vi "STAGE+mono+counter_edit19.vi"() -> ()   [LabVIEW 2017]
panel:
  out "PROGRESS":u8(slide) max=10 step=10 scale=0.0..100.0
  in  "?":enum32{"Page 1", "Page 2"}(tab)
  out "XY Graph":cluster{dbl[], dbl[]}(graph)
  out "XY Graph 2":cluster{dbl[], dbl[]}[](graph)
  in  "Collect Data!":bool
  out "Timeout":bool
  in  "?":bool
  out "Timeout 2":bool
  out "Waveform Graph":waveform(dbl)[](graph)
  in  "?":enum32{"DELAY", "COUNTER", "MONO", "PLOT"}(tab)
  out "Final time [ps]":dbl
  out "Current time [ps]":dbl
  out "Initial time [ps]":dbl
  in  "Set this as t0":bool
  in  "Axis":i32=1
  in  "Motor ON":bool
  in  "Motor OFF":bool
  out "Current Position [mm]":dbl
  out "Final Position [mm]":dbl
  in  "Data Points":i32=100
  out "Current Point":i32
  in  "Step Size [um]":i32=10
  in  "Target [mm]":dbl format="%.3f"
  in  "Move":bool
  out "Initial position [mm]":dbl
  in  "GPIB address":string="23"
  in  "Count Mode":u16(ring) items=["A,B for Preset T", "A-B for Preset T", "A+B for Preset T", "A for Preset B"]
  in  "Trigger mode":u16(ring) items=["10 MHz"=0, "Input 2"=2, "Input T"=3]
  in  "Channel A Input":u16(ring)=1 items=["10 MHz", "Input 1"]
  in  "Channel B Input":u16(ring)=2 items=["Input 1"=1, "Input 2"=2]
  in  "Number of Measurements\n to take at one point/ Number of Periods":u16=1 min=1 max=2000 step=1
  in  "Time between measurements\n at one point (s)/Dwell Time":dbl=0.002 min=0.002 max=60.0 step=0.001
  in  "gate mode (CW:0)":i16(slide) scale=0.0..2.0 scale format="%.2f"
  out "Counts":i32
  in  "Integrating time \nin 10^-7 sec":dbl=10000000.0
  in  "Discriminator Level (mV)":dbl min=-300.0 max=300.0 step=0.2
  in  "Discriminator Slope":bool
  in  "Channel":i16 min=0 max=2 step=1
  out "Grating #":dbl
  out "Blaze angle":dbl
  out "Grooves/mm":dbl
  out "Mono port":T1(ring)
  out "Time delay":u32=450000 min=1
  in  "Step size":dbl=10.0 min=0.0
  in  "Scan to":i32=4000
  in  "Scan from":i32=2600
  out "Current wavelength":dbl
  in  "?":bool
  in  "Array":dbl[](array[numeric])
  out "Numeric":i32
  out "Numeric 2":i32
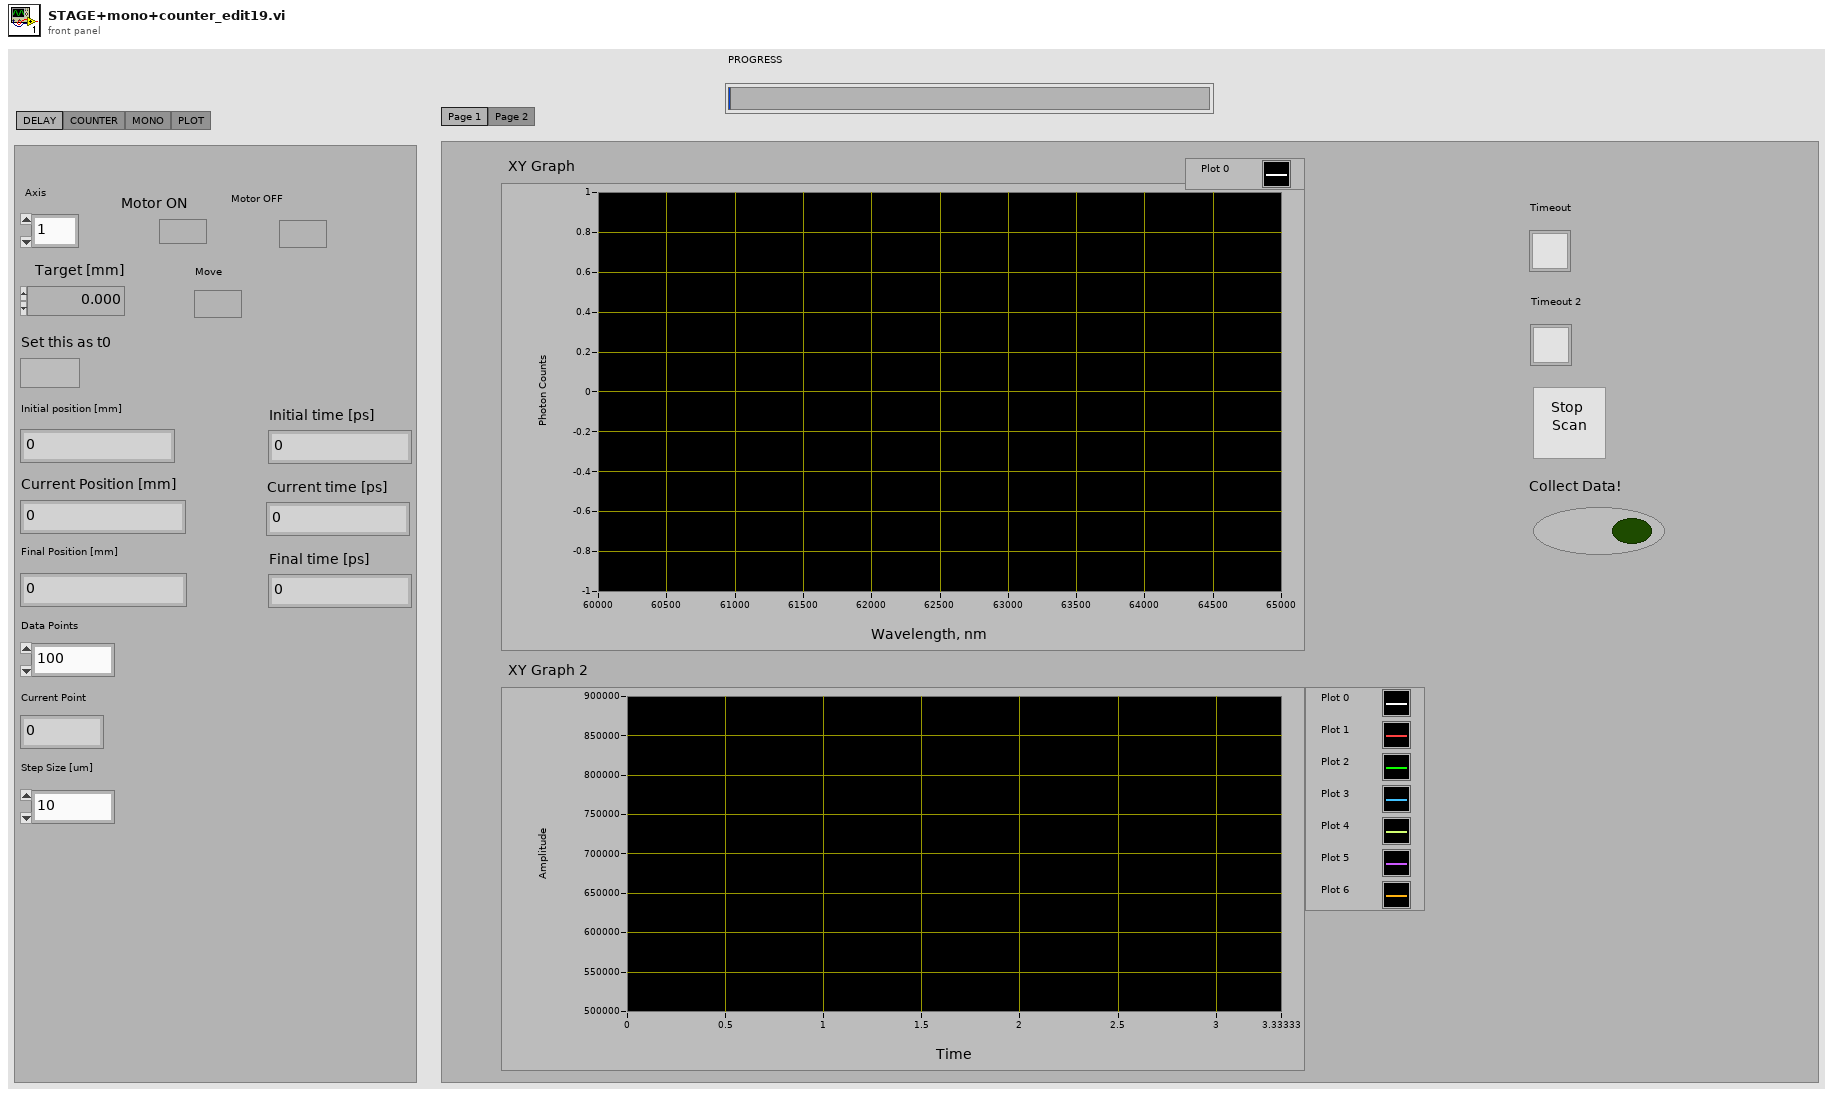
[diagram p1: front panel]
types:
  T1 = enum8{"COM 1", "COM 2", "COM 3", "COM 4", "COM 5", "COM 6", "COM 7", "COM 8", "COM 9"}
  T2 = cluster{"input XON/XOFF":bool, "input HW Handshake":bool, "input alt HW HShk":bool, "output XON/XOFF":bool, "output HW Handshake":bool, "output alt HW HShk":bool, "XOFF byte":u8, "XON byte":u8, "parity error byte":u16}
  T3 = enum16{"no parity", "odd parity", "even parity", "mark parity", "space parity"}
  T4 = typedef "NI_Matrix.lvlib/RealMatrix.ctl" = dbl[][]
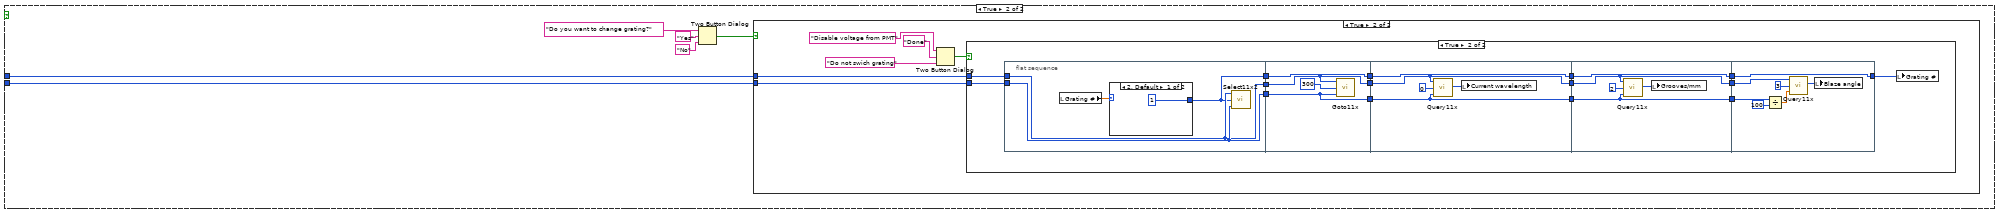
[diagram p2: hidden frame]
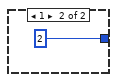
[diagram p5: hidden frame]
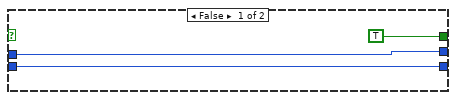
[diagram p6: hidden frame]
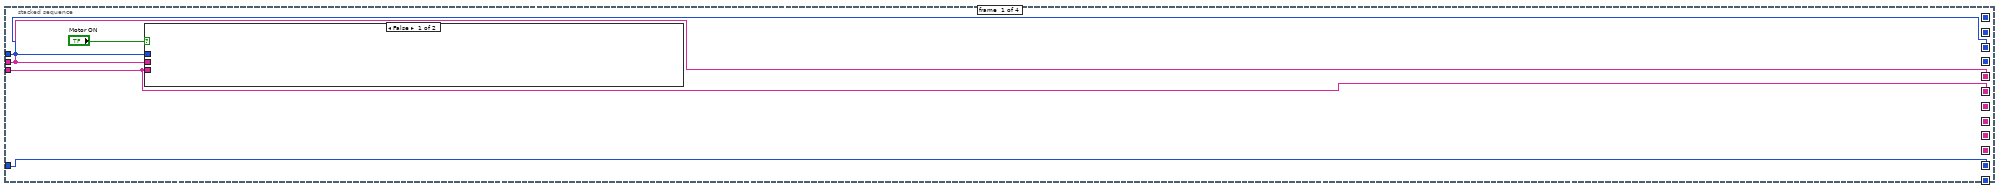
[diagram p7: hidden frame]
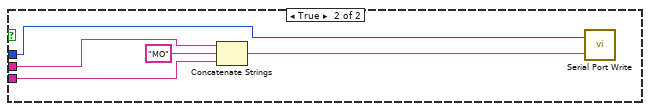
[diagram p8: hidden frame]
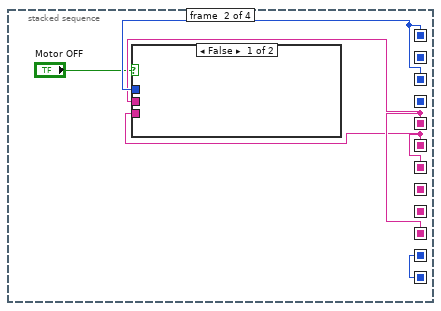
[diagram p9: hidden frame]
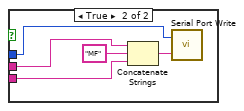
[diagram p10: hidden frame]
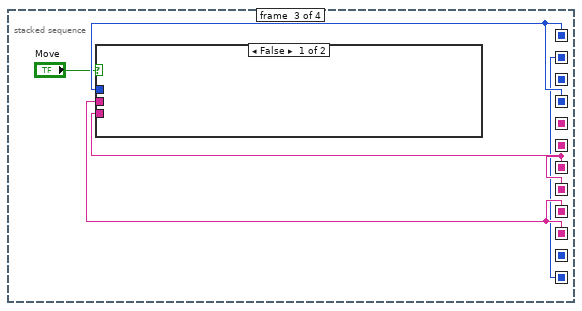
[diagram p11: hidden frame]
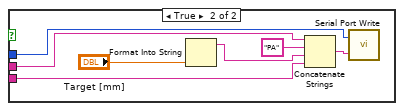
[diagram p12: hidden frame]
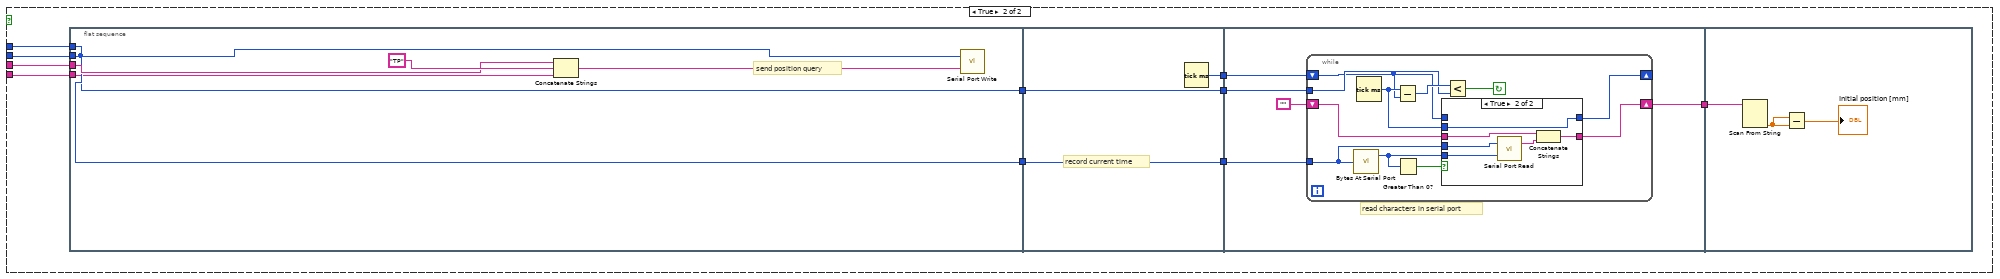
[diagram p13: hidden frame]
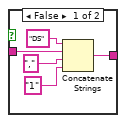
[diagram p15: hidden frame]
diagram:
  (unwired) FALSE
  w41 = u32 19200  # baud rate
  w40 = u16 8  # data bits
  w39 = enum16{"1 bit", "1.5 bits", "2 bits"}."1 bit"  # stop bits
  w43 = T3."no parity"  # parity
  w38 = 4  # 0=COM1 so n=COM(n+1)
  w42 = u16 1024  # buffer size
  n1 = flat-sequence {
    tunnel: ["Data Points"] -> w47
    tunnel: "Axis" -> [w69]
    tunnel: [w61] -> w46
    tunnel: [w69] -> w45
    tunnel: ["Step Size [um]"] -> w19
    tunnel: [w61] -> w18
    tunnel: ["Step Size [um]"] -> w17
    tunnel: ["Data Points"] -> w16
    tunnel: [w61] -> w15
    tunnel: [w60] -> w14
    tunnel: [w61] -> w12
    tunnel: [w60] -> w11
    tunnel: [w63] -> w10
    tunnel: [w52] -> w9
    tunnel: [w53] -> w2
    tunnel: [w52] -> w1
    tunnel: w47 -> [w161]
    tunnel: w46 -> [w160]
    tunnel: w45 -> [w159]
    tunnel: w38 -> [w155]
    tunnel: "GPIB address" -> [w154]
    tunnel: "GPIB address" -> [w153]
    tunnel: w19 -> [w142]
    tunnel: w18 -> [w140]
    tunnel: w17 -> [w139]
    tunnel: w16 -> [w137]
    tunnel: w15 -> [w132]
    tunnel: w14 -> [w131]
    tunnel: "Integrating time \nin 10^-7 sec" -> [w130]
    tunnel: w12 -> [w129]
    tunnel: w11 -> [w128]
    tunnel: w10 -> [w127]
    tunnel: w9 -> [w125]
    tunnel: w5 -> [w115]
    tunnel: w4 -> [w114]
    tunnel: w3 -> [w113]
    tunnel: w2 -> [w83]
    tunnel: w1 -> [w82]
    frame #0 {
      n2 = while {
        stop <- "Collect Data!" stop-if-true
        n3 = Multiply(x=1, y=1000) -> (x*y=w51:i32)
        n4 = Wait (ms)(milliseconds to wait=w51) -> ()  [unwired: 1 out]
      }
    }
    frame #1 {
      w54 = 1000000000000.0
      w59 = 1000
      w62 = 300000000
      w64 = 1000
      n5 = local read "Initial position [mm]"() -> (w61:dbl)
      n6 = Multiply(x="Step Size [um]", y="Data Points") -> (x*y=w68:i32)
      n7 = Divide(x=w68, y=w64) -> (x/y=w67:dbl)
      n8 = Divide(x="Step Size [um]", y=w64) -> (x/y=w63:dbl)
      n9 = Add(x=w61, y=w67) -> (x+y=w60:dbl)
      "Final Position [mm]" <- w60
      n10 = Divide(x=w60, y=w59) -> (x/y=w58:dbl)
      n11 = Divide(x=w61, y=w59) -> (x/y=w57:dbl)
      n12 = Divide(x=w58, y=w62) -> (x/y=w55:dbl)
      n13 = Divide(x=w57, y=w62) -> (x/y=w56:dbl)
      n14 = Multiply(x=w55, y=w54) -> (x*y=w53:dbl)
      "Final time [ps]" <- w53
      n15 = Multiply(x=w56, y=w54) -> (x*y=w52:dbl)
      "Initial time [ps]" <- w52
    }
    frame #2 {
      w74 = 1
      w95 = "\r\n"
      n16 = Increment(x=w137) -> (x+1=w138:i32)
      n17 = local read "Numeric 2"() -> (w78:i32)
      n18 = Multiply(x="Scan from", y=w74) -> (x*y=w70:i32)
      n19 = Multiply(x="Scan to", y=w74) -> (x*y=w72:i32)
      n20 = local read "Numeric"() -> (w77:i32)
      n21 = Divide(x=w142, y=1000.0) -> (x/y=w119:dbl)
      n22 = for {
        N: w138 -> [_]
        tunnel: w119 -> [w172]
        tunnel: w140 -> [w170]
        tunnel: [w163] -> w136 mode=indexing
        i -> [w171]
        # "distances"
        n23 = Multiply(x=w172, y=w171) -> (x*y=w169:dbl)
        n24 = Add(x=w170, y=w169) -> (x+y=w168:dbl)
        n25 = Divide(x=w168, y=1000) -> (x/y=w162:dbl)
        n26 = Divide(x=w162, y=300000000) -> (x/y=w165:dbl)
        n27 = Multiply(x=w165, y=1000000000000.0) -> (x*y=w163:dbl)
      }
      n28 = To Time Stamp(1:w70) -> (0:w86:timestamp)
      n29 = Initialize Array(0.0, w77, w78) -> ()  [unwired: 1 out]
      n30 = Multiply(x=w72, y=1) -> (x*y=w126:i32)
      n31 = Multiply(x=1, y=w70) -> (x*y=w118:i32)
      n32 = Divide(x=w119, y=1000.0) -> (x/y=w120:dbl)
      n33 = Subtract(x=w126, y=w118) -> (x-y=w148:i32)
      n34 = Divide(x=w120, y=300000000) -> (x/y=w122:dbl)
      n35 = Divide(x=w148, y="Step size") -> (x/y=w147:dbl)
      n36 = Bundle By Name("Y"=dbl[] [], "t0"=w86, "dt"="Step size") -> (w85:waveform(dbl))  [unwired: 1 in]
      n37 = property on="Waveform Graph" class="WFGraph (strict)"("XScale.Increment"="Step size", "XScale.Maximum"=w72, "XScale.Minimum"=w70) -> ()  [unwired: 2 in, 2 out]
      n38 = Multiply(x=w122, y=1000000000000.0) -> (x*y=w81:dbl)
      n39 = Build Array(w85) -> (w84:waveform(dbl)[])
      n40 = Round Toward -Infinity(1:w147) -> (0:w146:dbl)
      n41 = Concatenate Strings("\r", "\n") -> (w156:string)
      n42 = property on="XY Graph 2" class="XYGraph (strict)"("XScale.Increment"=w81, "XScale.Maximum"=w83, "XScale.Minimum"=w82) -> ()  [unwired: 2 in, 2 out]
      n43 = Increment(x=w146) -> (x+1=w117:dbl)
      n44 = for {
        N: w117 -> [_]
        tunnel: "Step size" -> [w177]
        tunnel: w118 -> [w175]
        tunnel: [w173] -> w116 mode=indexing
        i -> [w176]
        # "wavelengths"
        n45 = Multiply(x=w177, y=w176) -> (x*y=w174:dbl)
        n46 = Add(x=w175, y=w174) -> (x+y=w173:dbl)
      }
      n47 = for {
        N: w161 -> [w187]
        tunnel: w160 -> [w250]
        tunnel: w139 -> [w246]
        tunnel: w159 -> [w243]
        tunnel: w156 -> [w240]
        tunnel: w155 -> [w241]
        tunnel: w154 -> [w239]
        tunnel: w114 -> [w236]
        tunnel: w115 -> [w238]
        tunnel: w153 -> [w237]
        tunnel: [w197] -> w88 mode=indexing
        tunnel: w118 -> [w231]
        tunnel: "Step size" -> [w230]
        tunnel: w146 -> [w229]
        tunnel: w132 -> [_]
        tunnel: w131 -> [_]
        tunnel: w130 -> [w228]
        tunnel: w72 -> [w227]
        tunnel: w70 -> [w226]
        tunnel: "Step size" -> [w203]
        tunnel: w129 -> [w219]
        tunnel: w128 -> [w217]
        tunnel: w127 -> [w220]
        tunnel: w81 -> [w189]
        tunnel: w125 -> [w224]
        tunnel: w70 -> [w204]
        tunnel: "Step size" -> [w205]
        shift-right: [w188] -> _
        shift-left: dbl[] [] -> [w183]
        tunnel: w115 -> [w202]
        tunnel: w114 -> [w201]
        tunnel: w113 -> [w200]
        shift-right: [w194] -> _
        shift-left: w84 -> [w195]
        shift-right: [w181] -> _
        shift-left: dbl[][] [] -> [w180]
        i -> [w186]
        w199 = dbl[] []
        w218 = 1000
        w221 = 300000000
        n48 = To Time Stamp(1:w231) -> ()  [unwired: 1 out]
        n49 = stacked-sequence {
          tunnel: w236 -> [w461]
          tunnel: w237 -> [_]
          frame #0 {
            n50 = call <vilib>:"Close Serial Driver.vi"("port number"=w461) -> ()  [unwired: 1 out]
            n51 = GPIB Misc(0:"loc 23" ("command string")) -> ()  [unwired: 1 in, 3 out]
          }
        }
        n52 = property on="PROGRESS" class="Slide (strict)"("Scale.Increment"=1, "Scale.Maximum"=w187, "Scale.Minimum"=0) -> ()  [unwired: 2 in, 2 out]
        n53 = flat-sequence {
          tunnel: w239 -> [w276]
          tunnel: w238 -> [w275]
          tunnel: w236 -> [w274]
          tunnel: w231 -> [w273]
          tunnel: w230 -> [w272]
          tunnel: w229 -> [w271]
          tunnel: w227 -> [w270]
          tunnel: w226 -> [w269]
          tunnel: w199 -> [w268]
          tunnel: w199 -> [w267]
          tunnel: w205 -> [w266]
          tunnel: w204 -> [w265]
          tunnel: w203 -> [w264]
          tunnel: w202 -> [w263]
          tunnel: w201 -> [w262]
          tunnel: w200 -> [w261]
          tunnel: [w259] -> w198
          tunnel: [w260] -> _
          tunnel: [w259] -> w196
          tunnel: [w441] -> w197
          tunnel: w198 -> [w441]
          tunnel: [w440] -> w182
          tunnel: [w439] -> w179
          frame #0 {
            # "step size"
            n54 = while {
              tunnel: w274 -> [_]
              tunnel: w275 -> [_]
              tunnel: w276 -> [w282]
              tunnel: w273 -> [w310]
              tunnel: w272 -> [w309]
              tunnel: w271 -> [w308]
              tunnel: w270 -> [w278]
              tunnel: w269 -> [w277]
              tunnel: w264 -> [w279]
              tunnel: w266 -> [w306]
              shift-right: [w302] -> w259
              shift-left: w267 -> [w301]
              shift-right: [w296] -> w260
              shift-left: w268 -> [w304]
              tunnel: w265 -> [w299]
              tunnel: w263 -> [w286]
              tunnel: w262 -> [w285]
              tunnel: w261 -> [w284]
              i -> [w307]
              stop <- w313 stop-if-true
              n55 = property on="XY Graph" class="XYGraph (strict)"("XScale.Increment"=w279, "XScale.Maximum"=w278, "XScale.Minimum"=w277) -> ()  [unwired: 2 in, 2 out]
              n56 = Multiply(x=w307, y=w306) -> (x*y=w305:dbl)
              n57 = Multiply(x=w307, y=w309) -> (x*y=w314:dbl)
              n58 = Greater Or Equal?(x=w307, y=w308) -> (x >= y?=w311:bool)
              n59 = Add(x=w305, y=w299) -> ()  [unwired: 1 out]
              n60 = Add(x=w314, y=w310) -> (x+y=w283:dbl)
              n61 = Or(x="?", y=w311) -> (x .or. y?=w313:bool)
              n62 = Build Array (concatenate)(w304, w283) -> (w303:dbl[])
              n63 = flat-sequence {
                tunnel: w282 -> [w329]
                tunnel: w283 -> [w330]
                tunnel: [w330] -> w290
                tunnel: [w316] -> w289
                tunnel: [w315] -> w288
                tunnel: [w329] -> w287
                tunnel: w286 -> [w319]
                tunnel: w285 -> [w318]
                tunnel: w284 -> [w317]
                tunnel: [w363] -> w295
                tunnel: [w362] -> w294
                tunnel: [w360] -> w293
                tunnel: w290 -> [w364]
                tunnel: w289 -> [w363]
                tunnel: w288 -> [w362]
                tunnel: w287 -> [w360]
                tunnel: w295 -> [w371]
                tunnel: w294 -> [w370]
                tunnel: w293 -> [w365]
                tunnel: [w365] -> w281
                tunnel: w281 -> [w373]
                tunnel: [w373] -> w280
                tunnel: w280 -> [w426]
                tunnel: [w426] -> w292
                tunnel: w292 -> [w427]
                tunnel: [w427] -> w291
                tunnel: [w433] -> w298
                tunnel: w291 -> [w434]
                frame #0 {
                  n64 = flat-sequence {
                    tunnel: w319 -> [w336]
                    tunnel: [w336] -> w328
                    tunnel: w318 -> [w338]
                    tunnel: [w338] -> w327
                    tunnel: w317 -> [w334]
                    tunnel: [w334] -> w326
                    tunnel: w328 -> [w342]
                    tunnel: [w342] -> w325
                    tunnel: w327 -> [w343]
                    tunnel: [w343] -> w324
                    tunnel: w326 -> [w340]
                    tunnel: [w340] -> w323
                    tunnel: w325 -> [w351]
                    tunnel: [w351] -> w322
                    tunnel: w324 -> [w348]
                    tunnel: [w348] -> w321
                    tunnel: w323 -> [w346]
                    tunnel: [w346] -> w320
                    tunnel: w322 -> [w353]
                    tunnel: w321 -> [w354]
                    tunnel: w320 -> [_]
                    tunnel: [w354] -> w316
                    tunnel: [w353] -> w315
                    frame #0 {
                      n65 = call "Query11x.vi"("port number"=w338, "QUERY"=u16 0, "time delay"=w336) -> ("timeout"=w335:bool, "STATUS MESSAGE"=w333:u16)  [unwired: 2 out]
                      n66 = local write "Timeout"(w335) -> ()
                      n67 = Divide(x=w333, y=1 ("Numeric")) -> (x/y=→"Current wavelength":dbl)
                    }
                    frame #1 {
                      n68 = call "Query11x.vi"("port number"=w343, "QUERY"=u16 2, "time delay"=w342) -> ("timeout"=w341:bool, "STATUS MESSAGE"=→"Grooves/mm":u16)  [unwired: 2 out]
                      n69 = local write "Timeout"(w341) -> ()
                    }
                    frame #2 {
                      n70 = Divide(x=w351, y=i16 100 ("device (1)")) -> (x/y=w349:dbl)
                      n71 = call "Query11x.vi"("port number"=w348, "QUERY"=u16 3, "time delay"=w349) -> ("timeout"=w347:bool, "STATUS MESSAGE"=→"Blaze angle":u16)  [unwired: 2 out]
                      n72 = local write "Timeout"(w347) -> ()
                    }
                    frame #3 {
                      n73 = Divide(x=w353, y=i16 100 ("device (1)")) -> (x/y=w357:dbl)
                      n74 = call "Query11x.vi"("port number"=w354, "QUERY"=u16 4, "time delay"=w357) -> ("timeout"=w356:bool, "STATUS MESSAGE"=→"Grating #":u16)  [unwired: 2 out]
                      n75 = local write "Timeout"(w356) -> ()
                    }
                  }
                }
                frame #1 {
                  n76 = call "Goto11x.vi"("time delay"=w362, "WAVELENGTH"=w364, "port number"=w363) -> ("timeout"=w361:bool)  [unwired: 2 out]
                  n77 = local write "Timeout 2"(w361) -> ()
                }
                frame #2 {
                  # "set counter time in 10^-7 seconds in CW"
                  n78 = call "Query11x.vi"("port number"=w371, "QUERY"=0, "time delay"=w370) -> ("timeout"=w369:bool, "STATUS MESSAGE"=w368:u16)  [unwired: 2 out]
                  n79 = local write "Timeout 2"(w369) -> ()
                  n80 = Divide(x=w368, y=1) -> (x/y=w367:dbl)
                  n81 = local write "Current wavelength"(w367) -> ()
                }
                frame #3 {
                  # "Configures discriminator."
                  n82 = flat-sequence {
                    tunnel: w373 -> [w383]
                    tunnel: [w383] -> w382
                    tunnel: [w390] -> w381
                    tunnel: [w388] -> w380
                    tunnel: "Discriminator Slope" -> [w389]
                    tunnel: w382 -> [w388]
                    tunnel: w374 -> [w387]
                    tunnel: w381 -> [w409]
                    tunnel: [w410] -> w379
                    tunnel: w380 -> [w408]
                    tunnel: [w408] -> w378
                    tunnel: w374 -> [w406]
                    tunnel: w379 -> [w422]
                    tunnel: w378 -> [w421]
                    tunnel: "Discriminator Level (mV)" -> [w416]
                    tunnel: w374 -> [w415]
                    frame #0 {
                      # "Flush I/O buffers."
                      n83 = for {
                        N: 5 -> [_]
                        tunnel: w383 -> [w385]
                        n84 = GPIB Write(0:w385, 1:"\r") -> ()  [unwired: 3 in, 2 out]
                      }
                    }
                    frame #1 {
                      # "Set discriminator slope."
                      n85 = case shown="True" w389 {
                        tunnel: [w396 w401] -> w391
                        tunnel: w387 -> [w395 w400]
                        frame False {
                          n86 = Concatenate Strings("DS", w395, ",", "1") -> (w396:string)
                        }
                        frame True {
                          n87 = Concatenate Strings("DS", w400, ",", "0") -> (w401:string)
                        }
                      }
                      n88 = GPIB Write(0:w388, 1:w391, 2:5) -> (6:w390:errorcluster)  [unwired: 2 in, 1 out]
                    }
                    frame #2 {
                      # "Set discriminator mode to fixed."
                      n89 = Concatenate Strings("DM", w406, ",", "0") -> (w405:string)
                      n90 = GPIB Write(0:w408, 1:w405, 2:5, 3:w409) -> (6:w410:errorcluster)  [unwired: 1 in, 1 out]
                    }
                    frame #3 {
                      # "Set discriminator level.\nMust be between +300 and -300 mV."
                      n91 = Divide(x=w416, y=1000.0) -> (x/y=w424:dbl)
                      n92 = Number To Fractional String(number=w424, precision (6)=i16 4) -> (F-format string=w413:string)  [unwired: 2 in]
                      n93 = Concatenate Strings("DL", w415, ",", w413) -> (w420:string)
                      n94 = GPIB Write(0:w421, 1:w420, 2:5, 3:w422) -> (6:w417:errorcluster)  [unwired: 1 in, 1 out]
                      n95 = call <vilib>:"General Error Handler.vi"("type of dialog (OK msg:1)"=1, "error in (no error)"=w417) -> ()  [unwired: 9 in, 5 out]
                    }
                  }
                  n96 = Number To Decimal String(number="Channel") -> (decimal integer string=w374:string)  [unwired: 1 in]
                }
                frame #4 {
                  n97 = call "Start.vi"("GPIB Address"=w426) -> ()  [unwired: 9 in]
                }
                frame #5 {
                  # "Wait for Scan to Finish"
                  n98 = for {
                    N: 1 -> [_]
                    tunnel: w427 -> [w429]
                    n99 = while {
                      tunnel: w429 -> [w430]
                      stop <- w432 stop-if-true
                      n100 = call "ScanDone.vi"("Wait (ms)"=1000, "GPIB Address"=w430) -> ("Scan Finished?"=w432:bool)
                    }
                  }
                }
                frame #6 {
                  n101 = call "Read Data.vi"("Channel Number"=0, "GPIB Address"=w434, "Number of Datapoints"=1) -> ("Data"=w435:i32[])
                  n102 = Index Array(array=w435, index=0) -> (element=w433:i32)
                  "Counts" <- w433
                }
              }
              n103 = Build Array (concatenate)(w301, w298) -> (w300:dbl[])
              n104 = Bundle(w303, w300) -> (w297:cluster{dbl[], dbl[]})  [unwired: 1 in]
              "XY Graph" <- w297
              n105 = Unbundle(w297) -> (w296:dbl[], w302:dbl[])
            }
          }
          frame #1 {
            n106 = Array Size(array="Array") -> (size(s)=w439:i32)
            n107 = flat-sequence {
              tunnel: w441 -> [w447]
              tunnel: "Array" -> [w446]
              tunnel: w439 -> [w445]
              tunnel: [w443] -> w440
              frame #0 {
                n108 = for {
                  N: w445 -> [w452]
                  tunnel: w446 -> [w459]
                  tunnel: w447 -> [w454]
                  shift-right: [w448] -> w443
                  shift-left: dbl[] [] -> [w449]
                  i -> [w451]
                  n109 = local read "Scan from"() -> (w457:i32)
                  n110 = Index Array(array=w459, index=w451) -> (element=w458:dbl)
                  n111 = local read "Step size"() -> (w455:dbl)
                  n112 = Subtract(x=w458, y=w457) -> (x-y=w456:dbl)
                  n113 = Divide(x=w456, y=w455) -> (x/y=w453:dbl)
                  n114 = Index Array(array=w454, index=w453) -> (element=w450:dbl)
                  n115 = Insert Into Array(array=w449, index=w451, new element=w450) -> (w448:dbl[])
                  "Numeric" <- w452
                }
              }
            }
          }
        }
        n116 = Divide(x=w219, y=w218) -> (x/y=w215:dbl)
        n117 = Divide(x=w217, y=w218) -> (x/y=w214:dbl)
        n118 = Divide(x=w220, y=w218) -> (x/y=w216:dbl)
        n119 = Multiply(x=w189, y=w186) -> (x*y=w225:dbl)
        n120 = Number To Decimal String(number=w228) -> (decimal integer string=w234:string)  [unwired: 1 in]
        n121 = Add(x=1, y=w186) -> (x+y=→"PROGRESS":i32)
        n122 = Divide(x=w246, y=1000) -> (x/y=w245:dbl)
        n123 = Divide(x=w215, y=w221) -> (x/y=w209:dbl)
        n124 = Divide(x=w214, y=w221) -> (x/y=w208:dbl)
        n125 = Divide(x=w216, y=w221) -> (x/y=w210:dbl)
        n126 = Add(x=w224, y=w225) -> (x+y=w184:dbl)
        n127 = Concatenate Strings("CP 2,", w234) -> (w232:string)
        n128 = Multiply(x=w209, y=1000000000000.0) -> ()  [unwired: 1 out]
        n129 = Multiply(x=w208, y=1000000000000.0) -> ()  [unwired: 1 out]
        n130 = Multiply(x=w210, y=1000000000000.0) -> ()  [unwired: 1 out]
        n131 = Multiply(x=w245, y=w186) -> (x*y=w249:dbl)
        n132 = Build Array (concatenate)(w183, w184) -> (w185:dbl[])
        n133 = Add(x=w250, y=w249) -> (x+y=w248:dbl)
        n134 = Format Into String(w243) -> (resulting string=w242:string)  [unwired: 3 in, 1 out]
        n135 = GPIB Write(0:w239, 1:w232, 2:i16 5 ("mode (0)")) -> ()  [unwired: 2 in, 2 out]
        n136 = flat-sequence {
          tunnel: w248 -> [w464]
          tunnel: [w464] -> w244
          tunnel: w240 -> [w466]
          tunnel: w242 -> [w465]
          tunnel: w241 -> [w462]
          tunnel: w244 -> [w475]
          frame #0 {
            n137 = Format Into String(w464) -> (resulting string=w463:string)  [unwired: 3 in, 1 out]
            n138 = Wait (ms)(milliseconds to wait=u32 100) -> ()  [unwired: 1 out]
            n139 = Concatenate Strings(w465, "PA" ("Substring"), w463, w466) -> (w468:string)
            n140 = call <vilib>:"Serial Port Write.vi"("string to write"=w468, "port number"=w462) -> ()  [unwired: 1 out]
          }
          frame #1 {
            n141 = Divide(x=w475, y=1000) -> (x/y=w473:dbl)
            n142 = Wait (ms)(milliseconds to wait=u32 1000) -> ()  [unwired: 1 out]
            n143 = Divide(x=w473, y=300000000) -> (x/y=w472:dbl)
            n144 = Multiply(x=w472, y=1000000000000.0) -> (x*y=→"Current time [ps]":dbl)
            "Current Position [mm]" <- w475
          }
        }
        n145 = local read "Scan from"() -> (w192:i32)
        n146 = local read "Step size"() -> (w190:dbl)
        n147 = To Time Stamp(1:w192) -> (0:w191:timestamp)
        n148 = Bundle By Name("Y"=w196, "t0"=w191, "dt"=w190) -> (w193:waveform(dbl))  [unwired: 1 in]
        n149 = Build Array (concatenate)(w195, w193) -> (w194:waveform(dbl)[])
        "Waveform Graph" <- w194
        n150 = for {
          N: w179 -> [_]
          tunnel: [w258] -> w188
          tunnel: w185 -> [w257]
          tunnel: w182 -> [w255]
          tunnel: [w254] -> w181
          tunnel: w180 -> [w256]
          tunnel: [w251] -> w178 mode=indexing
          i -> [w253]
          n151 = Build Array (concatenate)(w256, w255) -> (w254:dbl[][])
          n152 = Index Array(array=w255, index=w253) -> ()  [unwired: 1 out]
          n153 = Index Array(array=w254, index (col)=w253) -> (element=w252:dbl[])  [unwired: 1 in]
          n154 = Bundle(w257, w252) -> (w251:cluster{dbl[], dbl[]})  [unwired: 1 in]
          n155 = Unbundle(w251) -> (w258:dbl[])  [unwired: 1 out]
        }
        "XY Graph 2" <- w178
        "Current Point" <- w186
        "Numeric 2" <- w187
      }
      n156 = Build Array (concatenate)(0, w136) -> (w89:dbl[])
      n157 = local read "Integrating time \nin 10^-7 sec"() -> (w93:dbl)
      n158 = Build Array(w116) -> (w145:dbl[][])
      n159 = Transpose Matrix(1:w145) -> (0:w144:dbl[][])
      n160 = Transpose Matrix(1:w88) -> (0:w143:dbl[][])
      n161 = Build Array (concatenate)(w144, w143) -> (w90:T4)
      n162 = Insert Into Array(array=w90, index (row)=0, new element=w89) -> (w133:T4)  [unwired: 1 in]
      n163 = local read "Blaze angle"() -> (w112:dbl)
      n164 = local read "Grating #"() -> (w111:dbl)
      n165 = Multiply(x=w93, y=1e-07) -> (x*y=w92:dbl)
      n166 = Get Date/Time In Seconds() -> (seconds since 1Jan1904=w105:timestamp)
      n167 = Array To Spreadsheet String(delimiter (Tab)=",", array=w133, 3:"%f" ("format string")) -> (spreadsheet string=w94:string)
      n168 = Format Date/Time String(time format string (%c)="%Y-%b-%d %H:%M:%S", seconds (now)=w105) -> (date/time string=w106:string)  [unwired: 1 in]
      n169 = Number To Decimal String(number=w92) -> (decimal integer string=w107:string)  [unwired: 1 in]
      n170 = Number To Decimal String(number=w111) -> (decimal integer string=w108:string)  [unwired: 1 in]
      n171 = Number To Decimal String(number=w112) -> (decimal integer string=w96:string)  [unwired: 1 in]
      n172 = call <vilib>:"Space Constant.vi"() -> ("String"=w109:string)
      n173 = Concatenate Strings(w95, "Data was taken on ", w106, w95, "Integration Time is ", w107, w109, "s", w95, "Monochromator gratng # ", w108, "; ", "blazed for ", w96, w109, "nm", w95, w95, w95, w94) -> (w110:string)
      n174 = Write to Text File(text=w110) -> ()  [unwired: 3 in, 3 out]
    }
  }
  n175 = flat-sequence {
    tunnel: [w479] -> w32
    tunnel: [w478] -> w31
    frame #0 {
      n176 = call "CM Com Read ini.vi"() -> ("Mono port"=w478:T1, "time delay1"=w479:u32)  [unwired: 7 in]
    }
  }
  n177 = call <vilib>:"Serial Port Init.vi"("flow control etc."=T2 {"input XON/XOFF"=FALSE, "input HW Handshake"=FALSE, "input alt HW HShk"=FALSE, "output XON/XOFF"=FALSE, "output HW Handshake"=FALSE, "output alt HW HShk"=FALSE, "XOFF byte"=13, "XON byte"=11, "parity error byte"=0}, "parity"=w43, "buffer size"=w42, "stop bits"=w39, "data bits"=w40, "baud rate"=w41, "port number"=w38) -> ("error code"=w37:i32)
  n178 = call "CM Serial Port Setup.vi"("COM port"=w31, "time delay"=w32) -> ("time delay1"=w27:u32, "DK port Out"=w28:T1, "error code"=w30:i32)  [unwired: 7 in]
  n179 = Equal To 0?(x=w30) -> (x = 0?=w29:bool)
  n180 = Concatenate Strings("\r", "\n") -> (w33:string)
  n181 = while {
    tunnel: w38 -> [w482]
    tunnel: w33 -> [w483]
    tunnel: w37 -> [_]
    tunnel: "Axis" -> [w480]
    stop <- TRUE continue-if-true
    w481 = u32 200  # timeout
    n182 = Format Into String(w480) -> (resulting string=w484:string)  [unwired: 3 in, 1 out]
    n183 = stacked-sequence {
      seq-local: [w489 _ _ _] -> [_ w500 _ _]
      seq-local: [w488 _ _ _] -> [_ w499 _ _]
      seq-local: [w490 _ _ _] -> [_ w501 _ _]
      seq-local: [w487 _ _ _] -> [_ w497 _ _]
      seq-local: [_ w500 _ _] -> [_ _ w510 _]
      seq-local: [_ w499 _ _] -> [_ _ w509 _]
      seq-local: [_ w501 _ _] -> [_ _ w511 _]
      seq-local: [_ w497 _ _] -> [_ _ w507 _]
      seq-local: [_ _ w510 _] -> [_ _ _ w523]
      seq-local: [_ _ w509 _] -> [_ _ _ w520]
      seq-local: [_ _ w511 _] -> [_ _ _ w522]
      seq-local: [_ _ w507 _] -> [_ _ _ w521]
      tunnel: w484 -> [w489 _ _ _]
      tunnel: w483 -> [w488 _ _ _]
      tunnel: w482 -> [w490 _ _ _]
      tunnel: w481 -> [w487 _ _ _]
      frame #0 {
        n184 = case shown="False" "Motor ON" {
          tunnel: w490 -> [_ w496]
          tunnel: w489 -> [_ w493]
          tunnel: w488 -> [_ w492]
          frame False {
          }
          frame True {
            n185 = Concatenate Strings(w493, "MO" ("Substring"), w492) -> (w494:string)
            n186 = call <vilib>:"Serial Port Write.vi"("string to write"=w494, "port number"=w496) -> ()  [unwired: 1 out]
          }
        }
      }
      frame #1 {
        n187 = case shown="False" "Motor OFF" {
          tunnel: w501 -> [_ w506]
          tunnel: w500 -> [_ w503]
          tunnel: w499 -> [_ w502]
          frame False {
          }
          frame True {
            n188 = Concatenate Strings(w503, "MF" ("Substring"), w502) -> (w504:string)
            n189 = call <vilib>:"Serial Port Write.vi"("string to write"=w504, "port number"=w506) -> ()  [unwired: 1 out]
          }
        }
      }
      frame #2 {
        n190 = case shown="False" "Move" {
          tunnel: w511 -> [_ w518]
          tunnel: w510 -> [_ w515]
          tunnel: w509 -> [_ w514]
          frame False {
          }
          frame True {
            n191 = Format Into String("Target [mm]") -> (resulting string=w512:string)  [unwired: 3 in, 1 out]
            n192 = Concatenate Strings(w515, "PA" ("Substring"), w512, w514) -> (w516:string)
            n193 = call <vilib>:"Serial Port Write.vi"("string to write"=w516, "port number"=w518) -> ()  [unwired: 1 out]
          }
        }
      }
      frame #3 {
        n194 = case shown="False" "Set this as t0" {
          tunnel: w523 -> [_ w533]
          tunnel: w522 -> [_ w532]
          tunnel: w521 -> [_ w531]
          tunnel: w520 -> [_ w530]
          frame False {
          }
          frame True {
            n195 = flat-sequence {
              tunnel: w533 -> [w537]
              tunnel: w532 -> [w536]
              tunnel: [w536] -> w529
              tunnel: w531 -> [w534]
              tunnel: [w534] -> w528
              tunnel: w530 -> [w535]
              tunnel: w529 -> [w541]
              tunnel: [w541] -> w527
              tunnel: w528 -> [w540]
              tunnel: [w540] -> w526
              tunnel: [w542] -> w525
              tunnel: w527 -> [w547]
              tunnel: w526 -> [w545]
              tunnel: w525 -> [w544]
              tunnel: [w543] -> w524
              tunnel: w524 -> [w569]
              frame #0 {
                # "send position query"
                n196 = Concatenate Strings(w537, "TP" ("Substring"), w535) -> (w538:string)
                n197 = call <vilib>:"Serial Port Write.vi"("string to write"=w538, "port number"=w536) -> ()  [unwired: 1 out]
              }
              frame #1 {
                # "record current time"
                n198 = Tick Count (ms)() -> (millisecond timer value=w542:u32)
              }
              frame #2 {
                # "read characters in serial port"
                n199 = while {
                  shift-left: w544 -> [w548]
                  shift-right: [w549] -> _
                  tunnel: w545 -> [w552]
                  shift-left: "" -> [w555]
                  shift-right: [w554] -> w543
                  tunnel: w547 -> [w556]
                  stop <- w551 continue-if-true
                  n200 = call <vilib>:"Bytes At Serial Port.vi"("port number"=w556) -> ("byte count"=w557:u32)  [unwired: 1 out]
                  n201 = Tick Count (ms)() -> (millisecond timer value=w550:u32)
                  n202 = Subtract(x=w550, y=w548) -> (x-y=w553:u32)
                  n203 = Greater Than 0?(x=w557) -> (x > 0?=w558:bool)
                  n204 = case shown="True" w558 {
                    tunnel: w557 -> [_ w566]
                    tunnel: w556 -> [_ w565]
                    tunnel: w555 -> [w560 w563]
                    tunnel: [w560 w562] -> w554
                    tunnel: [w559 w561] -> w549
                    tunnel: w550 -> [_ w561]
                    tunnel: w548 -> [w559 _]
                    frame False {
                    }
                    frame True {
                      n205 = call <vilib>:"Serial Port Read.vi"("requested byte count"=w566, "port number"=w565) -> ("string read"=w564:string)  [unwired: 1 out]
                      n206 = Concatenate Strings(w563, w564) -> (w562:string)
                    }
                  }
                  n207 = Less?(x=w553, y=w552) -> (x < y?=w551:bool)
                }
              }
              frame #3 {
                n208 = Scan From String(input string=w569) -> (output 1=w567:dbl)  [unwired: 4 in, 3 out]
                n209 = Subtract(x=w567, y=w567) -> (x-y=→"Initial position [mm]":dbl)
              }
            }
          }
        }
      }
    }
    n210 = Wait Until Next ms Multiple(millisecond multiple=u32 50) -> ()  [unwired: 1 out]
  }
  n211 = case shown="True" w29 {
    tunnel: w28 -> [w572 w575]
    tunnel: w27 -> [w571 w574]
    tunnel: [w572 w575] -> w4
    tunnel: [w571 w574] -> w5
    tunnel: [TRUE FALSE] -> w3
    frame False {
    }
    frame True {
      n212 = call "CM Com Write ini.vi"("time delay1"=w575, "Mono port"=w574) -> ()  [unwired: 7 in]
      n213 = local write "Mono port"(w575) -> ()
      n214 = local write "Time delay"(w574) -> ()
    }
  }
  n215 = case shown="False" "?" {
    tunnel: w5 -> [_ w577]
    tunnel: w4 -> [_ w576]
    frame False {
    }
    frame True {
      n216 = Two Button Dialog(message="Do you want to change grating?", 1:"No" ("F button name (\"Cancel\")"), 2:"Yes" ("T button name (\"OK\")")) -> (T button?=w578:bool)
      n217 = case shown="True" w578 {
        tunnel: w577 -> [_ w583]
        tunnel: w576 -> [_ w582]
        frame False {
        }
        frame True {
          n218 = Two Button Dialog(message="Disable voltage from PMT", 1:"Do not swich grating" ("F button name (\"Cancel\")"), 2:"Done" ("T button name (\"OK\")")) -> (T button?=w584:bool)
          n219 = case shown="True" w584 {
            tunnel: w583 -> [_ w602]
            tunnel: w582 -> [_ w601]
            frame False {
            }
            frame True {
              n220 = flat-sequence {
                tunnel: w602 -> [w606]
                tunnel: [w606] -> w599
                tunnel: w601 -> [w605]
                tunnel: [w605] -> w598
                tunnel: [w603] -> w597
                tunnel: w599 -> [w610]
                tunnel: [w610] -> w596
                tunnel: w598 -> [w611]
                tunnel: [w611] -> w595
                tunnel: w597 -> [w609]
                tunnel: [w609] -> w594
                tunnel: w596 -> [w617]
                tunnel: [w617] -> w593
                tunnel: w595 -> [w616]
                tunnel: [w616] -> w592
                tunnel: w594 -> [w614]
                tunnel: [w614] -> w591
                tunnel: w593 -> [w620]
                tunnel: [w620] -> w590
                tunnel: w592 -> [w621]
                tunnel: [w621] -> w589
                tunnel: w591 -> [w619]
                tunnel: [w619] -> w588
                tunnel: w590 -> [w625]
                tunnel: w589 -> [w626]
                tunnel: [w624] -> w600
                tunnel: w588 -> [w624]
                frame #0 {
                  n221 = local read "Grating #"() -> (w604:dbl)
                  n222 = case shown="2, Default" w604 {
                    tunnel: [1 2] -> w603
                    frame 2, Default {
                    }
                    frame 1 {
                    }
                  }
                  n223 = call "Select11x2.vi"("time delay"=w606, "NEW GRT?"=w603, "port number"=w605) -> ()  [unwired: 3 out]
                }
                frame #1 {
                  n224 = call "Goto11x.vi"("time delay"=w610, "WAVELENGTH"=u16 300, "port number"=w611) -> ()  [unwired: 3 out]
                }
                frame #2 {
                  n225 = call "Query11x.vi"("port number"=w616, "QUERY"=u16 0, "time delay"=w617) -> ("STATUS MESSAGE"=w613:u16)  [unwired: 3 out]
                  n226 = local write "Current wavelength"(w613) -> ()
                }
                frame #3 {
                  n227 = call "Query11x.vi"("port number"=w621, "QUERY"=u16 2, "time delay"=w620) -> ("STATUS MESSAGE"=w618:u16)  [unwired: 3 out]
                  n228 = local write "Grooves/mm"(w618) -> ()
                }
                frame #4 {
                  n229 = Divide(x=w625, y=i16 100 ("device (1)")) -> (x/y=w627:dbl)
                  n230 = call "Query11x.vi"("port number"=w626, "QUERY"=u16 3, "time delay"=w627) -> ("STATUS MESSAGE"=w623:u16)  [unwired: 3 out]
                  n231 = local write "Blaze angle"(w623) -> ()
                }
              }
              n232 = local write "Grating #"(w600) -> ()
            }
          }
        }
      }
    }
  }
  n233 = call "Configure.vi"("Dwell Time (s)"="Time between measurements\n at one point (s)/Dwell Time", "Channel T Input"="Trigger mode", "Channel B Input"="Channel B Input", "Channel A Input"="Channel A Input", "Integrating time, 10^-7 sec"="Integrating time \nin 10^-7 sec", "gate mode (CW:0)"="gate mode (CW:0)", "Scan End Mode"=FALSE, "Number of Periods"="Number of Measurements\n to take at one point/ Number of Periods", "Count Mode"="Count Mode", "GPIB Address"="GPIB address") -> ()
  "Mono port" <- w31
  "Time delay" <- w32
